vi "EOL CAN_Get_Motor_Position.vi"(11 "NetworkObjHandle":u32) -> (1 "Position":u8 format="%02x", 2 "TxRx Data":string[][](array[string]), 3 "Response Good?":bool)   [LabVIEW 2012]
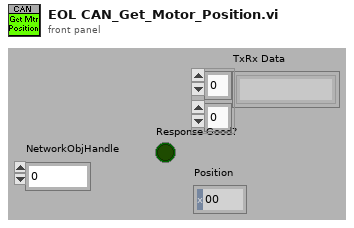
[diagram p1: front panel]
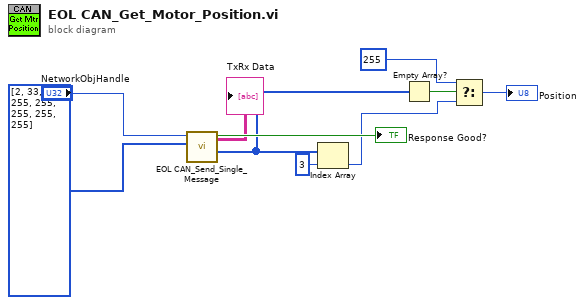
[diagram p0: block diagram]
diagram:
  n1 = call "EOL CAN_Send_Single_Message.vi"("Read Session in"=u8[] [2, 33, 64, 255, 255, 255, 255, 255] ("Transmit Data"), "Write Session in"="NetworkObjHandle") -> ("Rx Message"=w6:u8[], "Response Good?"=→"Response Good?":bool, "TxRx Data"=→"TxRx Data":string[][])  [unwired: 5 in, 2 out]
  n2 = Index Array(array=w6, index=3) -> (element=w3:u8)
  n3 = Empty Array?(array=w6) -> (empty?=w5:bool)
  n4 = Select(t=u8 255 ("CAN Data"), s=w5, f=w3) -> (s? t:f=→"Position":u8)
